vi "CallPython.vi"(8 "error in (no error)":errorcluster caption="Fehler (Eingang, kein Fehler)", 10 "command line":string="python HelloWorld.py", 11 "working directory":path=path "C:/apps/LabViewMeetsPython/Python") -> (0 "error out":errorcluster caption="Fehler (Ausgang)", 2 "standard output":string caption="Standardausgabe", 3 "return code":i32 caption="Fehlercode")   [LabVIEW 2013, in "CallPythonTools.lvlib"]
uses:
  CallPythonTools.lvlib
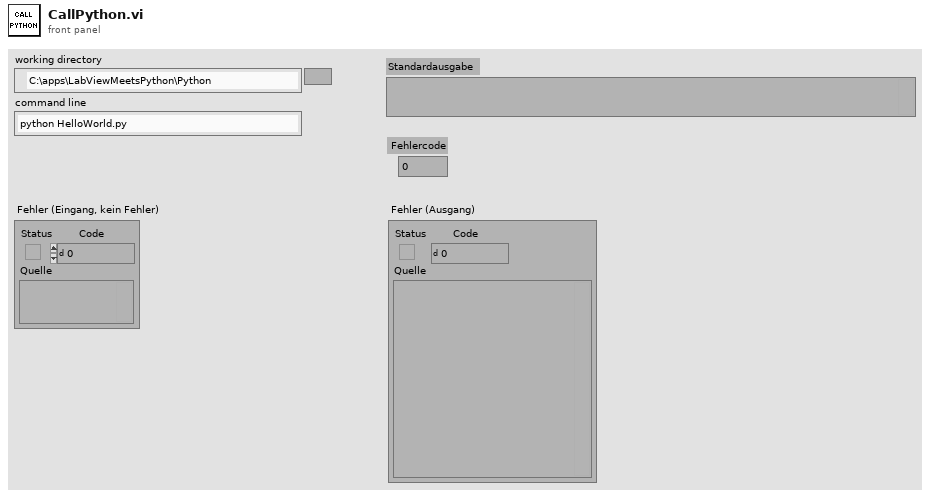
[diagram p1: front panel]
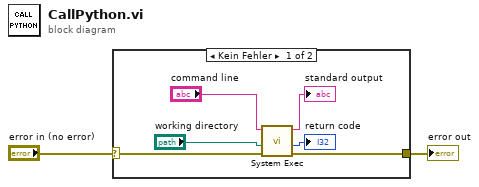
[diagram p0: block diagram]
diagram:
  n1 = case shown="Kein Fehler" "error in (no error)" {
    selector: "error in (no error)" -> [w3 w9]
    tunnel: [w4 w9] -> w1
    frame No Error {
      n2 = call <vilib>:"System Exec.vi"("error in (no error)"=w3, "working directory"="working directory", "command line"="command line") -> ("error out"=w4:errorcluster, "return code"=→"return code":i32, "standard output"=→"standard output":string)  [unwired: 5 in, 1 out]
    }
    frame Error {
    }
  }
  "error out" <- w1
